vi "svx_Autoscale Loose Fit.vi"(9 "Min":dbl, 11 "Max":dbl) -> (1 "Loose Fit Min":dbl, 3 "Loose Fit Max":dbl)   [LabVIEW 2017, in "SVX Waterfall Graph.xctl"]
uses:
  <vilib>/addons/_XControls/Waterfall Graph/SVX Waterfall Graph.xctl
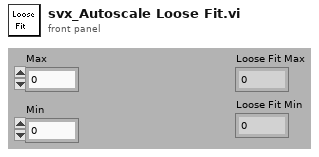
[diagram p1: front panel]
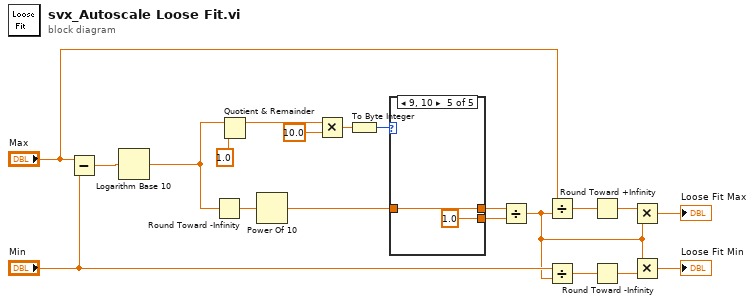
[diagram p0: block diagram]
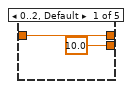
[diagram p2: hidden frame]
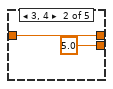
[diagram p3: hidden frame]
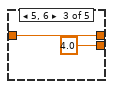
[diagram p4: hidden frame]
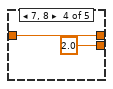
[diagram p5: hidden frame]
diagram:
  n1 = Subtract(x="Max", y="Min") -> (x-y=w10:dbl)
  n2 = Logarithm Base 10(1:w10) -> (0:w12:dbl)
  n3 = Round Toward -Infinity(1:w12) -> (0:w11:dbl)
  n4 = Quotient & Remainder(x=w12, y=1.0) -> (x-y*floor(x/y)=w14:dbl)  [unwired: 1 out]
  n5 = Power Of 10(x=w11) -> (10^x=w18:dbl)
  n6 = Multiply(x=w14, y=10.0) -> (x*y=w16:dbl)
  n7 = To Byte Integer(number=w16) -> (8bit integer=w17:i8)
  n8 = case shown="9, 10" w17 {
    tunnel: w18 -> [w22 w24 w26 w28 w30]
    tunnel: [w22 w24 w26 w28 w30] -> w19
    tunnel: [10.0 5.0 4.0 2.0 1.0] -> w20
    frame 0..2, Default {
    }
    frame 3, 4 {
    }
    frame 5, 6 {
    }
    frame 7, 8 {
    }
    frame 9, 10 {
    }
  }
  n9 = Divide(x=w19, y=w20) -> (x/y=w3:dbl)
  n10 = Divide(x="Max", y=w3) -> (x/y=w6:dbl)
  n11 = Divide(x="Min", y=w3) -> (x/y=w7:dbl)
  n12 = Round Toward +Infinity(x=w6) -> (ceil(x): smallest int >= x=w5:dbl)
  n13 = Round Toward -Infinity(1:w7) -> (0:w4:dbl)
  n14 = Multiply(x=w5, y=w3) -> (x*y=→"Loose Fit Max":dbl)
  n15 = Multiply(x=w3, y=w4) -> (x*y=→"Loose Fit Min":dbl)
